vi "Save Image.vi"(8 "error in (no error)":errorcluster, 10 "Path":path, 11 "Camera Controller in":refnum<class "Camera Controller.lvclass">) -> (0 "error out":errorcluster, 3 "Camera Controller out":refnum<class "Camera Controller.lvclass">)   [LabVIEW 2022 SP3, in "Camera Controller.lvclass"]
uses:
  Camera Controller.lvclass
  Camera Controller.lvclass/Camera Controller.ctl
  Camera Process Messages/Save Image Msg/Save Image Msg.lvclass
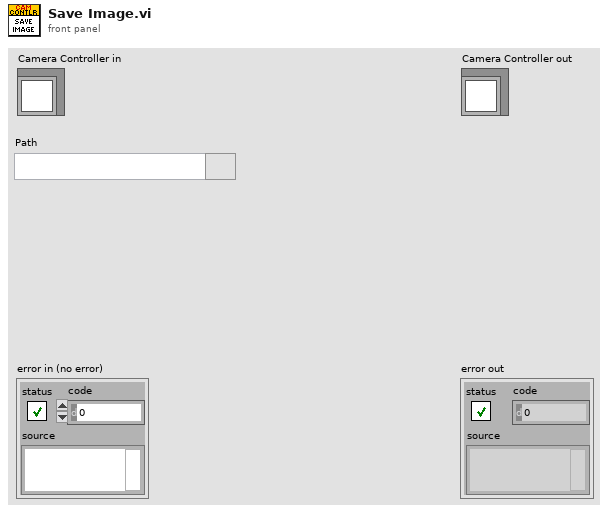
[diagram p1: front panel]
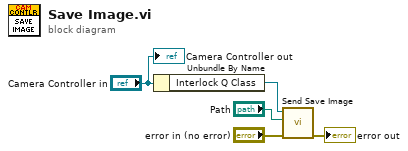
[diagram p0: block diagram]
diagram:
  n1 = Unbundle By Name("Camera Controller in") -> ("Interlock Q Class"=w4:refnum<class "Interlock Q Class.lvclass">)
  n2 = call "Send Save Image.vi"("error in (no error)"="error in (no error)", "Path"="Path", "Interlock Q Class in"=w4) -> ("error out"=→"error out":errorcluster)  [unwired: 7 in, 1 out]
  "Camera Controller out" <- "Camera Controller in"
